vi "zadanie4(SubVI).vi"(11 "read buffer":string) -> (3 "Numeric":dbl)   [LabVIEW 2019]
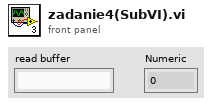
[diagram p1: front panel]
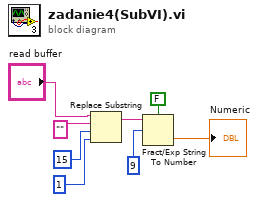
[diagram p0: block diagram]
diagram:
  n1 = Replace Substring(2:1 ("length (len. of substring)"), 3:15 ("offset (0)"), 4:"" ("substring (\"\")"), 5:"read buffer") -> (1:w8:string)  [unwired: 1 out]
  n2 = Fract/Exp String To Number(use system decimal point (T)=FALSE, string=w8, offset=9) -> (number=→"Numeric":dbl)  [unwired: 1 in, 1 out]
